vi "State_Machine.vi"(8 "error in (no error)":errorcluster caption="entrée d'erreur (pas d'erreur)", 11 "Get_Voltage en entrée":refnum<class "P2056_Send_Command_UART.lvclass">) -> (0 "error out":errorcluster caption="sortie d'erreur", 2 "Json_String":string, 3 "Get_Voltage en sortie":refnum<class "P2056_Send_Command_UART.lvclass">)   [LabVIEW 2020, in "Library Test.lvlib" / "P2056_Send_Command_UART.lvclass"]
uses:
  P2056_Send_Command_UART.lvclass
  C:/Users/ngarcin/OneDrive - Altyor/Standard TB/Class/Test/Test (Default)/Test (Default).lvclass
  JSON API/Variant JSON/Variant to JSON.vi
  JSON API/JSON Value/Get Item by name array.vi
  Instrument/Instrument (Default)/Class Instrument (Default).lvclass
  JSON API/JSON Value/JSON Value.lvclass
  P2056_Send_Command_UART.lvclass/P2056_Send_Command_UART.ctl
  JSON API/Get Polymorphic/JSON GetSet.lvlib
  JSON API/Variant JSON/Variant JSON.lvlib
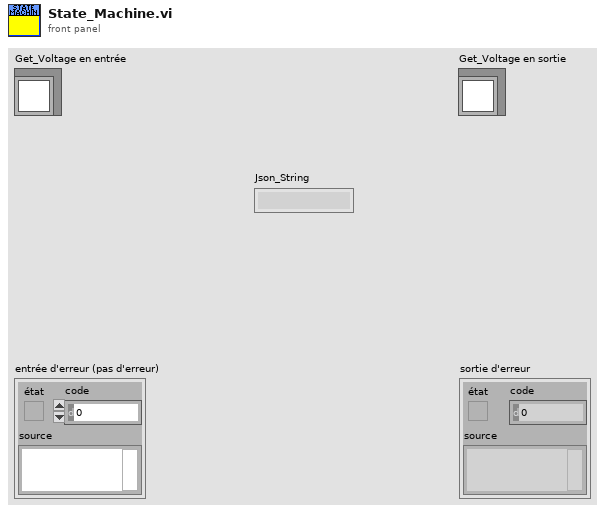
[diagram p1: front panel]
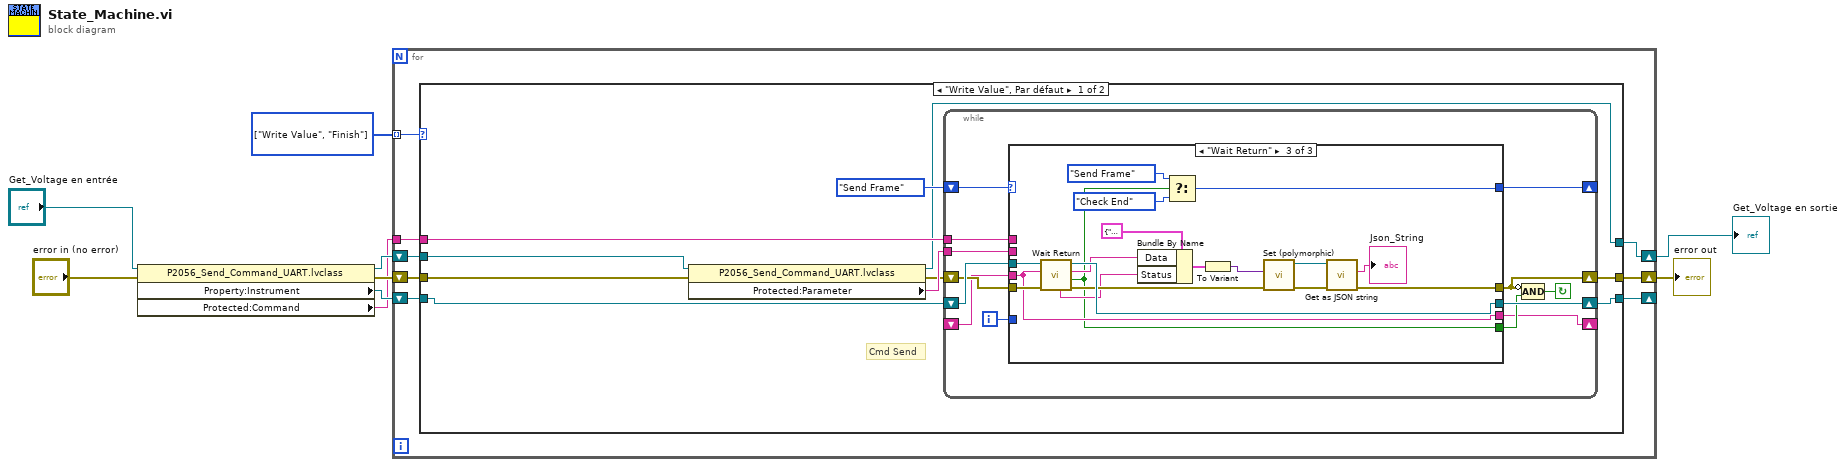
[diagram p0: block diagram]
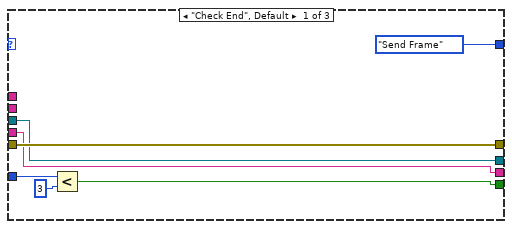
[diagram p2: hidden frame]
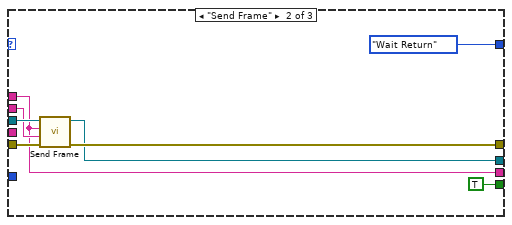
[diagram p3: hidden frame]
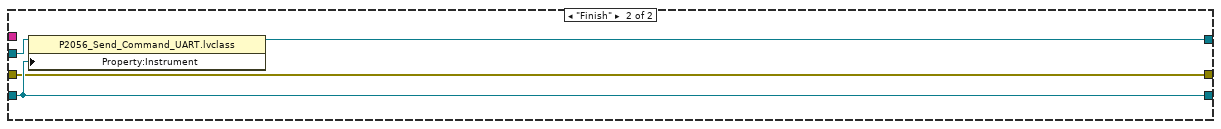
[diagram p4: hidden frame]
diagram:
  w6 = enum16{"Init", "Write Value", "Finish"}[] [enum."Write Value", enum."Finish"] items=["Init", "Write Value", "Finish"]
  n1 = property class="P2056_Send_Command_UART.lvclass"(reference="Get_Voltage en entrée", error in="error in (no error)") -> (reference out=w4:refnum<class "P2056_Send_Command_UART.lvclass">, error out=w3:errorcluster, "Property:Instrument"=w5:refnum<class "Class Instrument (Default).lvclass">, "Protected:Command"=w1:string)
  n2 = for {
    tunnel: w6 -> [w17] mode=indexing
    shift-right: [w15] -> _
    shift-left: w5 -> [w16]
    shift-right: [w13] -> w7
    shift-left: w4 -> [w14]
    shift-right: [w11] -> w8
    shift-left: w3 -> [w12]
    tunnel: w1 -> [w10]
    n3 = case shown="\"Write Value\", Par défaut" w17 {
      tunnel: w16 -> [w24 w75]
      tunnel: [w26 w75] -> w15
      tunnel: w14 -> [w22 w77]
      tunnel: [w21 w76] -> w13
      tunnel: w12 -> [w19 w74]
      tunnel: [w27 w74] -> w11
      tunnel: w10 -> [w25 _]
      frame "Write Value", Default {
        # "Cmd Send"
        n4 = property class="P2056_Send_Command_UART.lvclass"(reference=w22, error in=w19) -> (reference out=w21:refnum<class "P2056_Send_Command_UART.lvclass">, error out=w18:errorcluster, "Protected:Parameter"=w20:string)
        n5 = while {
          tunnel: w25 -> [w39]
          shift-right: [w40] -> w26
          shift-left: w24 -> [w38]
          shift-right: [w31] -> w27
          shift-left: w18 -> [w37]
          shift-right: [w36] -> _
          shift-left: enum16{"Send Frame", "Wait Return", "Check End"}."Send Frame" -> [w35]
          shift-right: [w28] -> _
          shift-left: _ -> [w34]
          tunnel: w20 -> [w33]
          i -> [w32]
          stop <- w29 continue-if-true
          n6 = case shown="\"Wait Return\"" w35 {
            tunnel: [w46 w55 w63] -> w31
            tunnel: [w45 w54 w71] -> w40
            tunnel: w39 -> [_ w48 _]
            tunnel: w38 -> [w45 w53 w72]
            tunnel: w37 -> [w46 w52 w73]
            tunnel: [enum16{"Send Frame", "Wait Return", "Check End"}."Send Frame" enum16{"Send Frame", "Wait Return", "Check End"}."Wait Return" w69] -> w36
            tunnel: [w41 TRUE ("Frame NOk") w56] -> w30
            tunnel: [w44 w48 w62] -> w28
            tunnel: w34 -> [w44 _ w62]
            tunnel: w33 -> [_ w49 _]
            tunnel: w32 -> [w42 _ _]
            frame "Check End", Default {
              n7 = Less?(x=w42, y=3) -> (x < y?=w41:bool)
            }
            frame "Send Frame" {
              n8 = call "Send Frame.vi"("entrée d'erreur (pas d'erreur)"=w52, "Parameter"=w49, "Cmd"=w48, "Class Instrument (Default) en entrée"=w53) -> ("sortie d'erreur"=w55:errorcluster, "Class Instrument (Default) en sortie"=w54:refnum<class "Class Instrument (Default).lvclass">)  [unwired: 6 in]
            }
            frame "Wait Return" {
              n9 = call "Wait Return.vi"("entrée d'erreur (pas d'erreur)"=w73, "Property:Data en entrée"=w62, "Class Instrument (Default) en entrée"=w72) -> ("sortie d'erreur"=w64:errorcluster, "Return"=w56:bool, "Data"=w59:string, "Class Instrument (Default) en sortie"=w71:refnum<class "Class Instrument (Default).lvclass">, "Status"=w58:string)  [unwired: 4 in]
              n10 = Bundle By Name(cluster=cluster{"Data":string, "Status":string} {"Data"="", "Status"=""}, "Data"=w59, "Status"=w58) -> (w57:cluster{"Data":string, "Status":string})
              n11 = Select(t=enum16{"Send Frame", "Wait Return", "Check End"}."Send Frame", s=w56, f=enum16{"Send Frame", "Wait Return", "Check End"}."Check End") -> (s? t:f=w69:enum16{"Send Frame", "Wait Return", "Check End"})
              n12 = To Variant(anything=w57) -> (Variant=w67:variant)
              n13 = call-poly "Set (polymorphic).vi"("error in (no error)"=w64, "Variant"=w67) -> ("error out"=w65:errorcluster, "JSON Value out"=w66:refnum<class "JSON Value.lvclass">)  [unwired: 8 in]
              n14 = call "Get as JSON string.vi"("error in (no error)"=w65, "JSON Value in"=w66) -> ("error out"=w63:errorcluster, "<JSON>"=→"Json_String":string)  [unwired: 8 in]
            }
          }
          n15 = Compound Arithmetic op=AND(invert w31, w30) -> (w29:bool)
        }
      }
      frame "Finish" {
        n16 = property class="P2056_Send_Command_UART.lvclass"(reference=w77, "Property:Instrument"=w75) -> (reference out=w76:refnum<class "P2056_Send_Command_UART.lvclass">)  [unwired: 1 in, 1 out]
      }
    }
  }
  "error out" <- w8
  "Get_Voltage en sortie" <- w7
